vi "histograms.vi"(0 "Host Plot Controls":T1={"refresh"=FALSE, "PMTs for Host"={"Sa"=0, "Sb"=1, "g-factor"=1}, "Peaks"={"# bins"=1000, "min"=0.020751953125, "max"=0.00103759765625}, "Averages"={"# bins"=1000, "max"=0.020751953125, "min"=0.00103759765625}, "Durations"={"# bins"=1000, "max"=20.0, "min"=8.0}, "FP-FPGA"={"# bins"=1000, "max"=20.0, "min"=8.0}, "FP-Host"={"# bins"=1000, "max"=20.0, "min"=8.0}, "Max or Average"=0} {"Max or Average" items=["Peak Max", "Peak Average"]}, 4 "peaks data":T3, 7 "?":T2) -> (16 "Number of drops detected":i32, 21 "H(peaks) vs peaks [volts]":cluster{"Axis":dbl[], i32[]}[](graph), 22 "H(durations) vs. durations [ms]":cluster{"Axis":dbl[], i32[]}(graph), 27 "?":T2)   [LabVIEW 2009]
uses:
  <vilib>/Analysis/NI_AALPro.lvlib
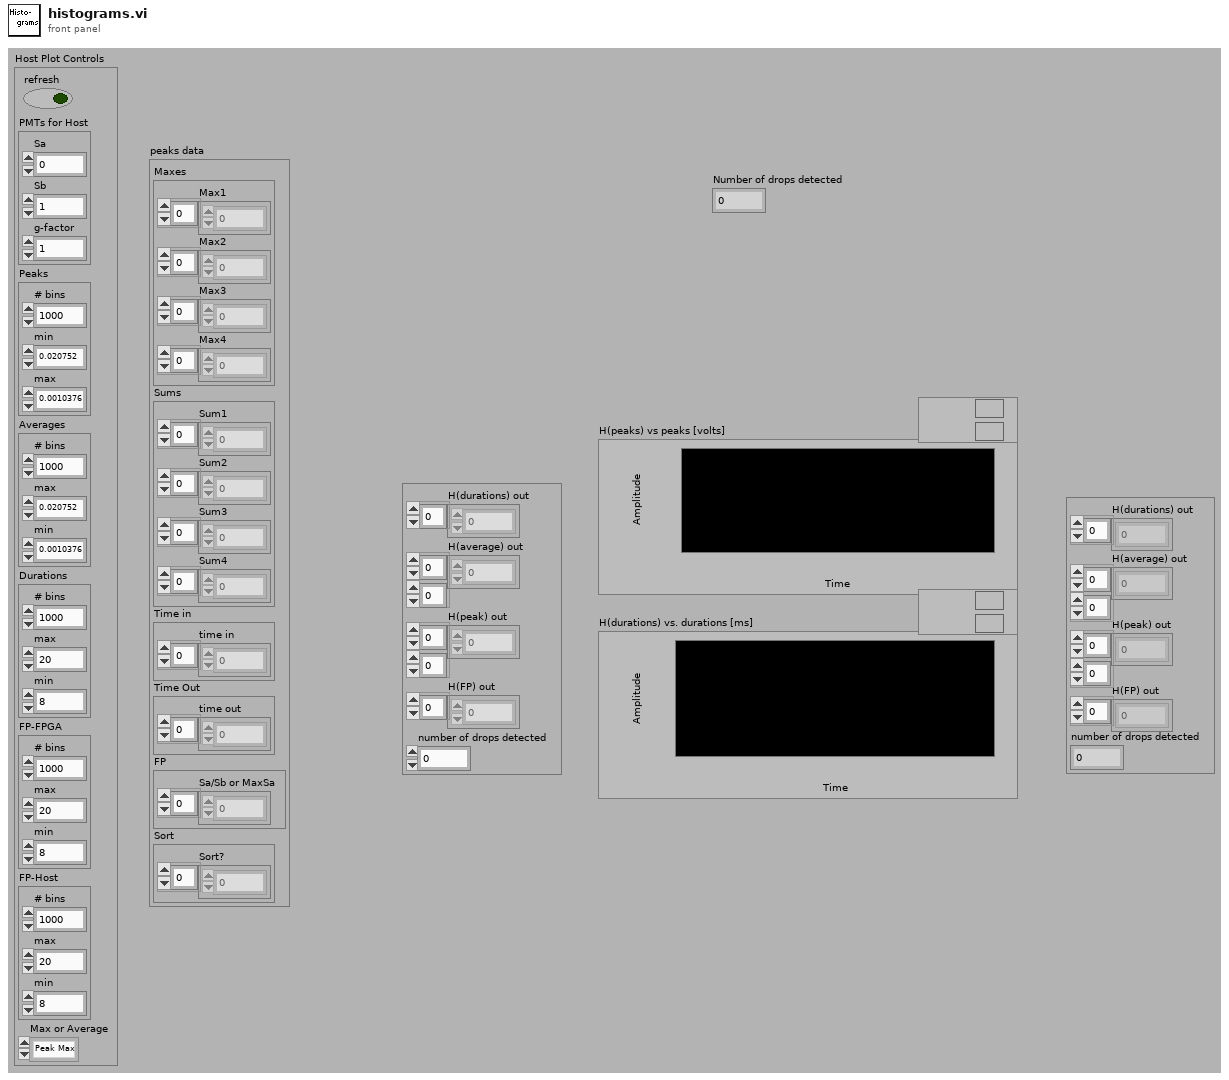
[diagram p1: front panel]
types:
  T1 = cluster{"refresh":bool, "PMTs for Host":cluster{"Sa":i8, "Sb":i8, "g-factor":i32}, "Peaks":cluster{"# bins":i32, "min":dbl, "max":dbl}, "Averages":cluster{"# bins":i32, "max":dbl, "min":dbl}, "Durations":cluster{"# bins":i32, "max":dbl, "min":dbl}, "FP-FPGA":cluster{"# bins":i32, "max":dbl, "min":dbl}, "FP-Host":cluster{"# bins":i32, "max":dbl, "min":dbl}, "Max or Average":i8}
  T2 = cluster{"H(durations) out":i32[], "H(average) out":i32[][], "H(peak) out":i32[][], "H(FP) out":i32[], "number of drops detected":i32}
  T3 = cluster{"Maxes":cluster{"Max1":dbl[], "Max2":dbl[], "Max3":dbl[], "Max4":dbl[]}, "Sums":cluster{"Sum1":dbl[], "Sum2":dbl[], "Sum3":dbl[], "Sum4":dbl[]}, "Time in":cluster{"time in":dbl[]}, "Time Out":cluster{"time out":dbl[]}, "FP":cluster{"Sa/Sb or MaxSa":dbl[]}, "Sort":cluster{"Sort?":dbl[]}}
  T4 = cluster{"Sum1":dbl[], "Sum2":dbl[], "Sum3":dbl[], "Sum4":dbl[]}
  T5 = cluster{"Max1":dbl[], "Max2":dbl[], "Max3":dbl[], "Max4":dbl[]}
  T6 = cluster{"H(durations) out":i32[], "H(peak) out":i32[][], "H(peak) out":i32[][], "H(durations) out":i32[], i32}
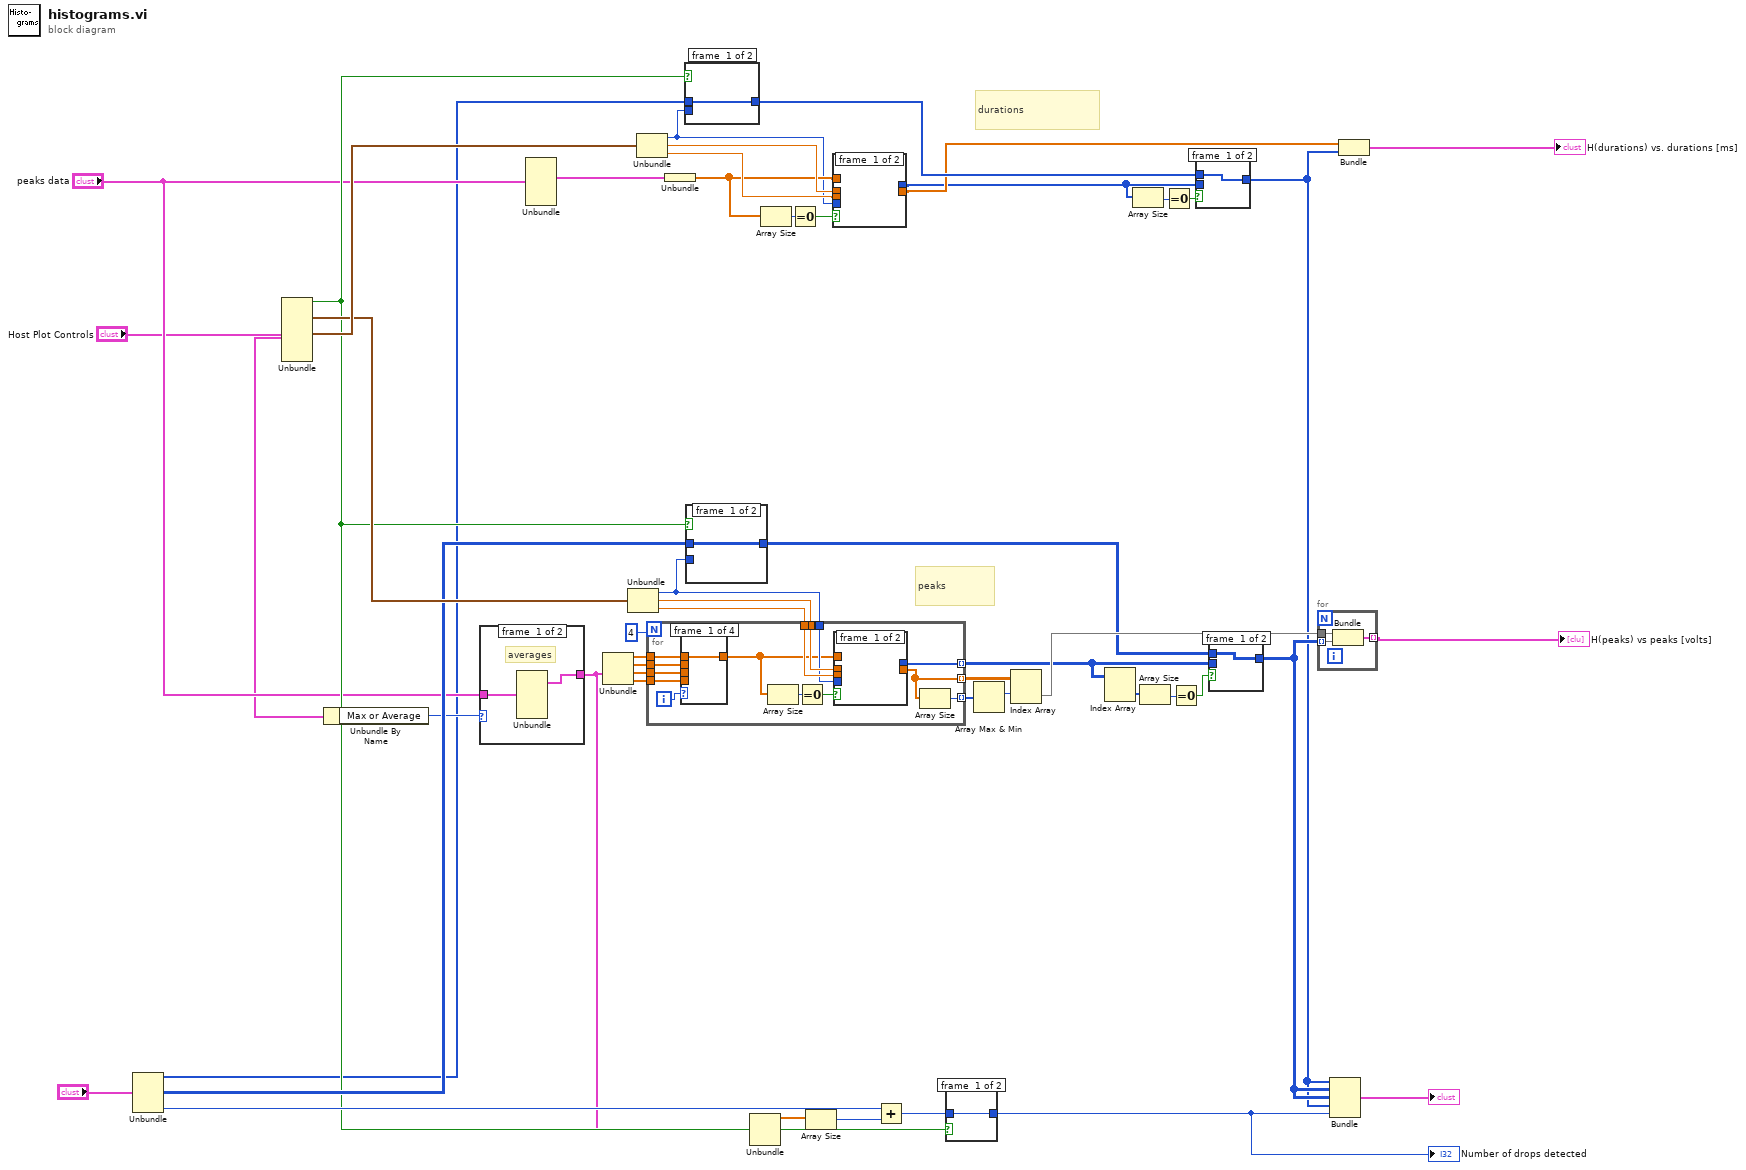
[diagram p0: block diagram]
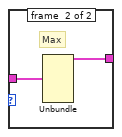
[diagram p2: hidden frame]
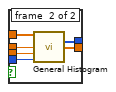
[diagram p3: hidden frame]
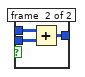
[diagram p4: hidden frame]
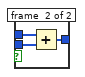
[diagram p5: hidden frame]
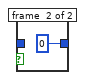
[diagram p6: hidden frame]
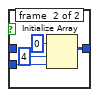
[diagram p7: hidden frame]
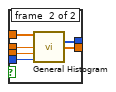
[diagram p8: hidden frame]
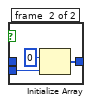
[diagram p12: hidden frame]
diagram:
  # "peaks"
  # "durations"
  n1 = Unbundle("?") -> ("H(durations) out"=w1:i32[], "H(peak) out"=w29:i32[][], "number of drops detected"=w28:i32)  [unwired: 2 out]
  n2 = Unbundle("Host Plot Controls") -> ("refresh"=w17:bool, "Peaks"=w30:cluster{"# bins":i32, "min":dbl, "max":dbl}, "Durations"=w44:cluster{"# bins":i32, "max":dbl, "min":dbl})  [unwired: 5 out]
  n3 = Unbundle By Name("Host Plot Controls") -> ("Max or Average"=w5:i8)
  n4 = case shown="1" w5 {
    tunnel: "peaks data" -> [w51 w53]
    tunnel: [w50 w52] -> w4
    frame #0 {
      # "averages"
      n5 = Unbundle(w51) -> ("Sums"=w50:T4)  [unwired: 5 out]
    }
    frame #1 {
      # "Max"
      n6 = Unbundle(w53) -> ("Maxes"=w52:T5)  [unwired: 5 out]
    }
  }
  n7 = Unbundle("peaks data") -> ("Time in"=w46:cluster{"time in":dbl[]})  [unwired: 5 out]
  n8 = Unbundle(w4) -> ("Max1"=w39:dbl[], "Max2"=w38:dbl[], "Max3"=w37:dbl[], "Max4"=w36:dbl[])
  n9 = Unbundle(w30) -> ("# bins"=w43:i32, "min"=w41:dbl, "max"=w42:dbl)
  n10 = Unbundle(w44) -> ("# bins"=w11:i32, "max"=w15:dbl, "min"=w14:dbl)
  n11 = for {
    N: 4 -> [_]
    tunnel: w39 -> [w66]
    tunnel: w38 -> [w65]
    tunnel: w37 -> [w64]
    tunnel: w36 -> [w63]
    tunnel: [w62] -> w20 mode=indexing
    tunnel: [w61] -> w34 mode=indexing
    tunnel: [w60] -> w33 mode=indexing
    tunnel: w41 -> [w59]
    tunnel: w42 -> [w58]
    tunnel: w43 -> [w57]
    i -> [w67]
    n12 = case shown="3" w67 {
      tunnel: w66 -> [w74 _ _ _]
      tunnel: w65 -> [_ w75 _ _]
      tunnel: w64 -> [_ _ w76 _]
      tunnel: w63 -> [_ _ _ w77]
      tunnel: [w74 w75 w76 w77] -> w56
      frame #0 {
      }
      frame #1 {
      }
      frame #2 {
      }
      frame #3 {
      }
    }
    n13 = Array Size(array=w56) -> (size(s)=w55:i32)
    n14 = Equal To 0?(x=w55) -> (x = 0?=w54:bool)
    n15 = case shown="False" w54 {
      tunnel: [_ w73] -> w62
      tunnel: [_ w72] -> w60
      tunnel: w56 -> [_ w71]
      tunnel: w59 -> [_ w70]
      tunnel: w58 -> [_ w69]
      tunnel: w57 -> [_ w68]
      frame #0 {
      }
      frame #1 {
        n16 = call <vilib>:"General Histogram.vi"("X"=w71, "max"=w70, "min"=w69, "# bins"=w68) -> ("Histogram"=w73:i32[], "Axis"=w72:dbl[])  [unwired: 7 in, 3 out]
      }
    }
    n17 = Array Size(array=w60) -> (size(s)=w61:i32)
  }
  n18 = Unbundle(w46) -> ("time in"=w12:dbl[])
  n19 = case shown="True" w17 {
    tunnel: [w78 w80] -> w45
    tunnel: w11 -> [_ w79]
    tunnel: w1 -> [w78 _]
    frame #0 {
    }
    frame #1 {
      n20 = Initialize Array(0, w79) -> (w80:i32[])
    }
  }
  n21 = case shown="True" w17 {
    tunnel: [w82 w85] -> w19
    tunnel: w43 -> [_ w84]
    tunnel: w29 -> [w82 _]
    frame #0 {
    }
    frame #1 {
      n22 = Initialize Array(0, 4, w84) -> (w85:i32[][])
    }
  }
  n23 = Unbundle(w4) -> ("Max1"=w8:dbl[])  [unwired: 3 out]
  n24 = Array Size(array=w12) -> (size(s)=w16:i32)
  n25 = Equal To 0?(x=w16) -> (x = 0?=w13:bool)
  n26 = Array Size(array=w8) -> (size(s)=w48:i32)
  n27 = case shown="False" w13 {
    tunnel: [_ w92] -> w9
    tunnel: [_ w91] -> w10
    tunnel: w12 -> [_ w90]
    tunnel: w15 -> [_ w89]
    tunnel: w14 -> [_ w88]
    tunnel: w11 -> [_ w87]
    frame #0 {
    }
    frame #1 {
      n28 = call <vilib>:"General Histogram.vi"("X"=w90, "max"=w89, "min"=w88, "# bins"=w87) -> ("Histogram"=w92:i32[], "Axis"=w91:dbl[])  [unwired: 7 in, 3 out]
    }
  }
  n29 = Add(x=w28, y=w48) -> (x+y=w27:i32)
  n30 = case shown="True" w17 {
    tunnel: w27 -> [w93 _]
    tunnel: [w93 0] -> w26
    frame #0 {
    }
    frame #1 {
    }
  }
  "Number of drops detected" <- w26
  n31 = Array Max & Min(array=w34) -> (max index (indices)=w32:i32)  [unwired: 3 out]
  n32 = Index Array(array=w33, index (row)=w32) -> (element=w40:dbl[])  [unwired: 1 in]
  n33 = Index Array(array=w20) -> (element=w23:i32[])  [unwired: 2 in]
  n34 = Array Size(array=w9) -> (size(s)=w25:i32)
  n35 = Array Size(array=w23) -> (size(s)=w22:i32)
  n36 = Equal To 0?(x=w25) -> (x = 0?=w24:bool)
  n37 = Equal To 0?(x=w22) -> (x = 0?=w21:bool)
  n38 = case shown="False" w24 {
    tunnel: [w95 w98] -> w6
    tunnel: w45 -> [w95 w97]
    tunnel: w9 -> [_ w96]
    frame #0 {
    }
    frame #1 {
      n39 = Add(x=w97, y=w96) -> (x+y=w98:i32[])
    }
  }
  n40 = case shown="False" w21 {
    tunnel: [w99 w102] -> w7
    tunnel: w19 -> [w99 w101]
    tunnel: w20 -> [_ w100]
    frame #0 {
    }
    frame #1 {
      n41 = Add(x=w101, y=w100) -> (x+y=w102:i32[][])
    }
  }
  n42 = for {
    tunnel: w40 -> [w105]
    tunnel: w7 -> [w104] mode=indexing
    tunnel: [w103] -> w31 mode=indexing
    n43 = Bundle("Axis"=w105, "H(peak) out"=w104) -> (w103:cluster{"Axis":dbl[], "H(peak) out":i32[]})  [unwired: 1 in]
  }
  "H(peaks) vs peaks [volts]" <- w31
  n44 = Bundle("H(durations) out"=w6, "H(peak) out"=w7, "H(peak) out"=w7, "H(durations) out"=w6, w26) -> (→"?":T6)  [unwired: 1 in]
  n45 = Bundle("Axis"=w10, "H(durations) out"=w6) -> (→"H(durations) vs. durations [ms]":cluster{"Axis":dbl[], "H(durations) out":i32[]})  [unwired: 1 in]
